vi "RichToFlatni_protobuf_types_DoubleAnalogWaveform.vi"(5 "OutputClusterType":T1, 11 "InputCluster":T5) -> (3 "OutputCluster":T1)   [LabVIEW 2021, in "ni.protobuf.types.lvlib"]
uses:
  ni.protobuf.types.lvlib
  ni_protobuf_types_DoubleAnalogWaveform.ctl
  ni_protobuf_types_PrecisionTimestamp.ctl
  ni_protobuf_types_DoubleAnalogWaveform_AttributesEntry.ctl
  ni_protobuf_types_WaveformAttributeValue_attribute/ni_protobuf_types_WaveformAttributeValue_attribute.lvclass
  ni_protobuf_types_WaveformAttributeValue.ctl
  ni_protobuf_types_DoubleAnalogWaveform_Flat.ctl
  ni_protobuf_types_PrecisionTimestamp_Flat.ctl
  ni_protobuf_types_DoubleAnalogWaveform_AttributesEntry_Flat.ctl
  ni_protobuf_types_WaveformAttributeValue_Flat.ctl
  ni_protobuf_types_WaveformAttributeValue_attribute/ni_protobuf_types_WaveformAttributeValue_attribute.lvclass/ni_protobuf_types_WaveformAttributeValue_attribute.ctl
  RichToFlatni_protobuf_types_WaveformAttributeValue.vi
  ni_protobuf_types_WaveformAttributeValue_attribute/GetActiveFieldIndex.vi
  ni_protobuf_types_WaveformAttributeValue_attribute/Getbool_value.vi
  ni_protobuf_types_WaveformAttributeValue_attribute/Getinteger_value.vi
  ni_protobuf_types_WaveformAttributeValue_attribute/Getdouble_value.vi
  ni_protobuf_types_WaveformAttributeValue_attribute/Getstring_value.vi
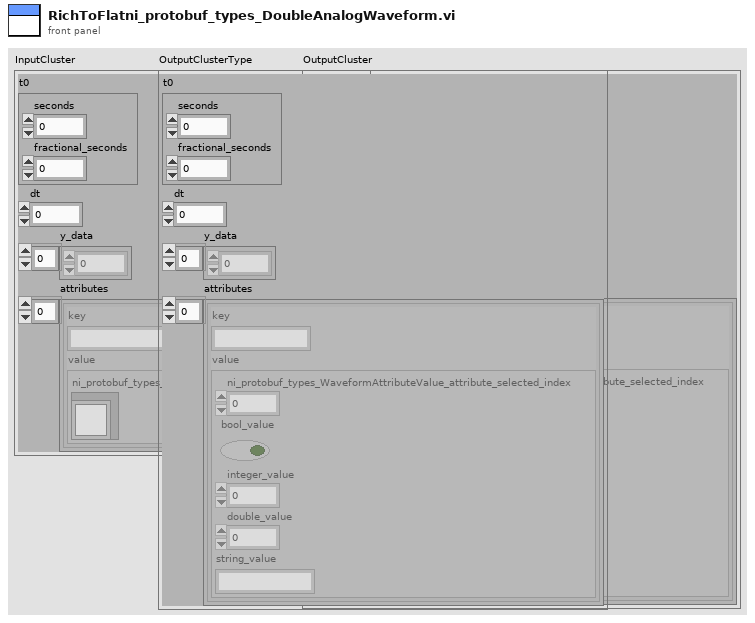
[diagram p1: front panel]
types:
  T1 = typedef "ni.protobuf.types.lvlib/ni_protobuf_types_DoubleAnalogWaveform_Flat.ctl" = cluster{"t0":T2, "dt":dbl, "y_data":dbl[], "attributes":T3[]}
  T2 = typedef "ni.protobuf.types.lvlib/ni_protobuf_types_PrecisionTimestamp_Flat.ctl" = cluster{"seconds":i64, "fractional_seconds":u64}
  T3 = typedef "ni.protobuf.types.lvlib/ni_protobuf_types_DoubleAnalogWaveform_AttributesEntry_Flat.ctl" = cluster{"key":string, "value":T4}
  T4 = typedef "ni.protobuf.types.lvlib/ni_protobuf_types_WaveformAttributeValue_Flat.ctl" = cluster{"ni_protobuf_types_WaveformAttributeValue_attribute_selected_index":i32, "bool_value":bool, "integer_value":i32, "double_value":dbl, "string_value":string}
  T5 = typedef "ni.protobuf.types.lvlib/ni_protobuf_types_DoubleAnalogWaveform.ctl" = cluster{"t0":T6, "dt":dbl, "y_data":dbl[], "attributes":T7[]}
  T6 = typedef "ni.protobuf.types.lvlib/ni_protobuf_types_PrecisionTimestamp.ctl" = cluster{"seconds":i64, "fractional_seconds":u64}
  T7 = typedef "ni.protobuf.types.lvlib/ni_protobuf_types_DoubleAnalogWaveform_AttributesEntry.ctl" = cluster{"key":string, "value":T8}
  T8 = typedef "ni.protobuf.types.lvlib/ni_protobuf_types_WaveformAttributeValue.ctl" = cluster{"ni_protobuf_types_WaveformAttributeValue_attribute":refnum<class "ni_protobuf_types_WaveformAttributeValue_attribute.lvclass">}
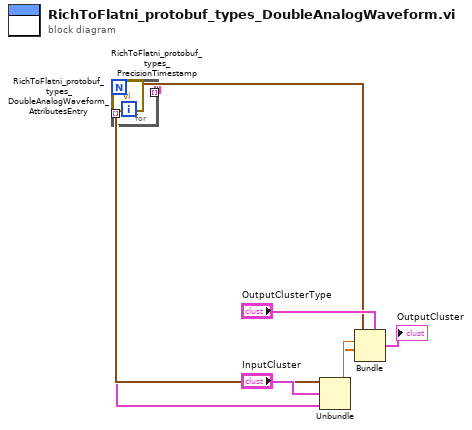
[diagram p0: block diagram]
diagram:
  n1 = Unbundle "Unbundle"("InputCluster") -> ("t0"=w6:T6, "dt"=w4:dbl, "y_data"=w3:dbl[], "attributes"=w2:T7[])
  n2 = for {
    tunnel: w2 -> [w11] mode=indexing
    tunnel: [w10] -> w1 mode=indexing
    n3 = call "RichToFlatni_protobuf_types_DoubleAnalogWaveform_AttributesEntry.vi"("InputCluster"=w11) -> ("OutputCluster"=w10:T3)  [unwired: 10 in]
  }
  n4 = call "RichToFlatni_protobuf_types_PrecisionTimestamp.vi"("InputCluster"=w6) -> ("OutputCluster"=w5:T2)  [unwired: 10 in]
  n5 = Bundle "Bundle"(cluster="OutputClusterType", "t0"=w5, "dt"=w4, "y_data"=w3, "attributes"=w1) -> (→"OutputCluster":T1)
